vi "Current Waveform Editor.vi"() -> ()   [LabVIEW 2017]
uses:
  <vilib>/Waveform/WDTOps.llb/WDT Append Waveforms DBL.vi
  <vilib>/Waveform/WDTFileIO.llb/ Write Waveform to File.vi
  <vilib>/Waveform/WDTOps.llb/WDT Waveform Duration DBL.vi
panel:
  in  "Load 4":bool
  out "Estimate Time 2":dbl caption="Estimate Time" format="%#_4p (H)"
  out "Estimate Time":dbl format="%#_4p (H)"
  in  "Battery":dbl=310.0 format="%#_6p(mAh)"
  out "Max 3":dbl
  out "Record#":i32
  out "dt":dbl
  out "File_duration(s)":dbl
  in  "Load_Org":bool
  out "Min_F_File":dbl
  out "Max_F_FILE":dbl
  out "Min":dbl
  out "Max":dbl
  out "Min File":path
  out "Max_file":path
  out "Total Samples (20KS)":dbl format="%#_9g"
  out "Total_Duration":dbl
  out "X2_FILE#":dbl
  out "X1_FILE#":dbl
  out "#WF IN File":i32[](array[numeric])
  out "X2_20KS_FILE#":dbl
  out "X1_20KS_FILE#":dbl
  out "X2_20KS":dbl
  out "X1_20KS":dbl
  out "Duration":dbl
  out "File_list":path[](array[path])
  in  "Load 3":bool
  out "Loop ?":i32
  out "selected path 2":path caption="selected path"
  out "selected path":path
  out "Sample Rate 2":dbl caption="Sample Rate" format="%#.6pS/s"
  in  "Load 2":bool
  out "Waveform_main 2":waveform(dbl)(graph)
  out "Avg (mA) 2":dbl caption="Avg (mA)"
  out "Minutes 2":u32 caption="Total Time" format="%<%H:%M:%S>t"
  in  "Save 2":bool
  in  "Center 2":bool
  in  "ZOOM M1M2 2":bool
  in  "Clear Graph 2":bool
  out "Min 2":dbl
  in  "Orginal 2":bool
  out "Total Time":u32 format="%<%H:%M:%S>t"
  out "Avg (mA)":dbl
  out "Sample Rate":dbl format="%#.6pS/s"
  in  "Save":bool
  in  "Load":bool
  in  "Orginal":bool
  in  "Clear Graph":bool
  in  "ZOOM M1M2":bool
  in  "stop":bool
  in  "Center":bool
  out "Waveform_main":waveform(dbl)(graph)
  out "Boolean":bool
  in  "uA_bank0":dbl=1.5 format="%#_13g"
  # "Current Waveform Editor V1.0"
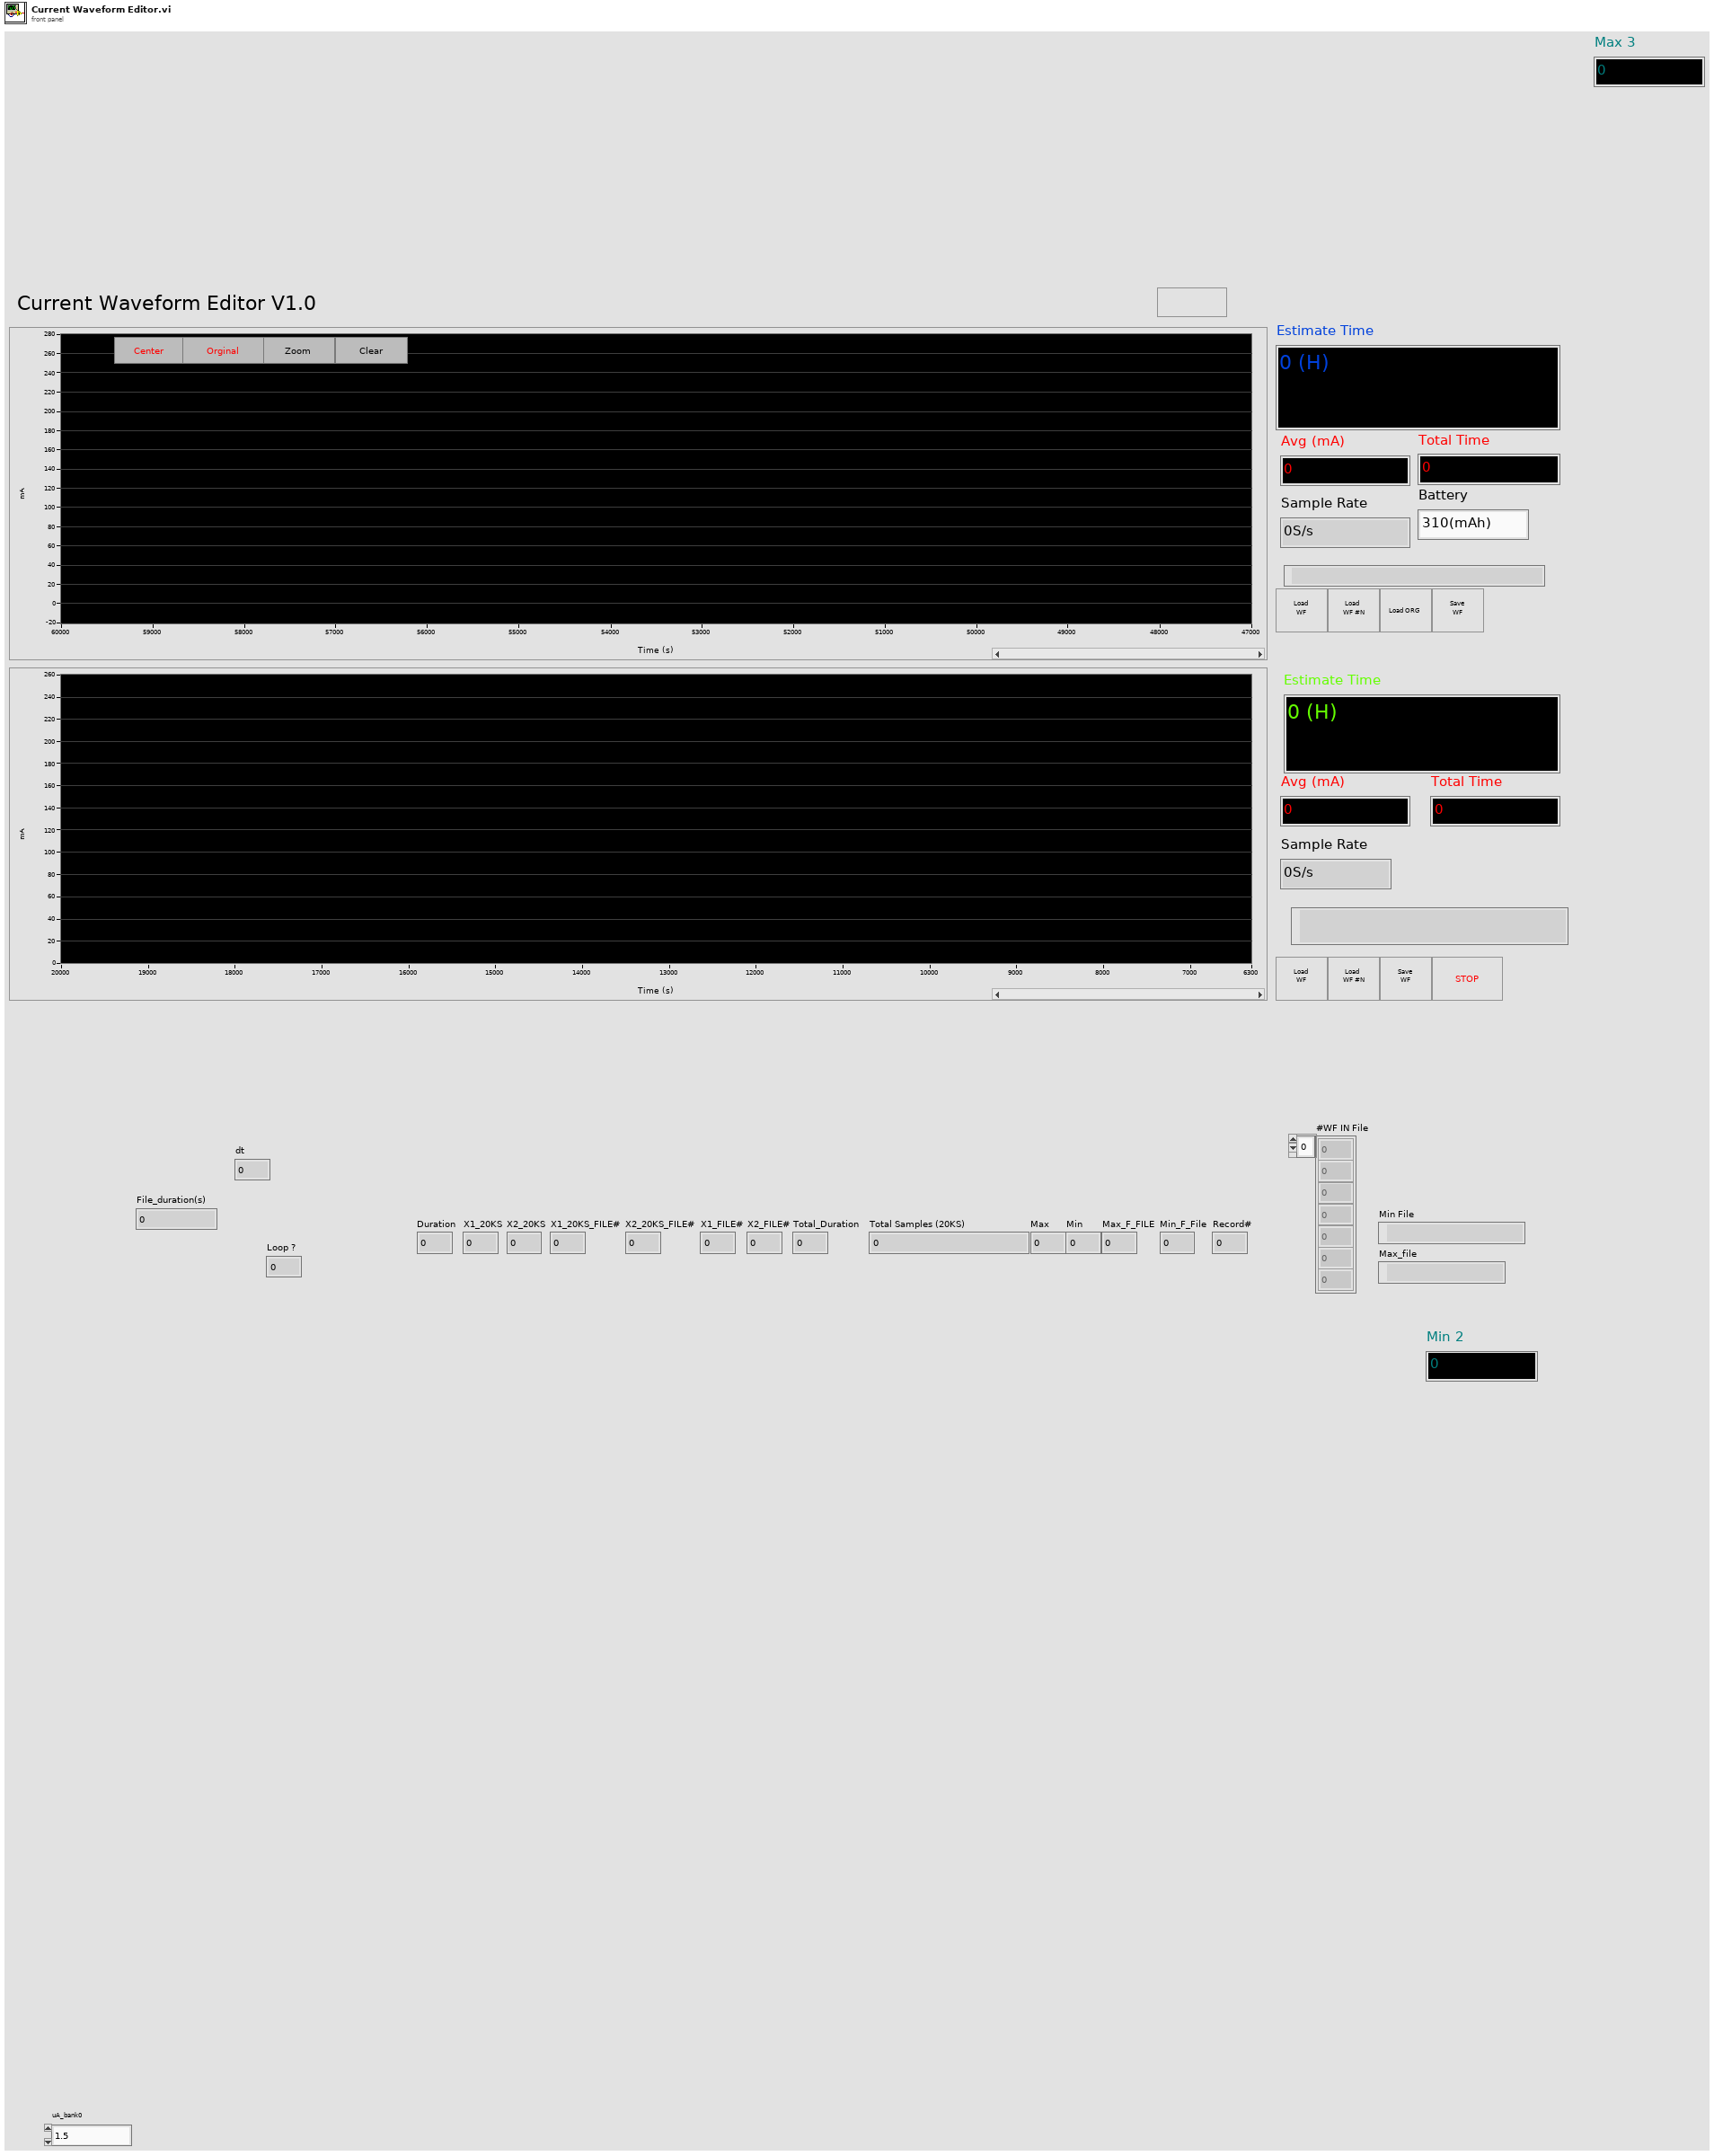
[diagram p1: front panel]
types:
  T1 = typedef "LVCursorListTypeDef.ctl" = cluster{"Name":string, "Color":u32, "Style":u8, "Point Style":u8, "Name Visible":bool, "Allow Drag":bool, "Cursor Mode":u32, "Plot":i32, "Index":i32, "Position":cluster{"X":dbl, "Y":dbl}, "X Scale":u32, "Y Scale":u32, "Watch Plots":i32[], "Watch All Plots":bool, "Plot Area":i32, "Label Offset":cluster{"X":dbl, "Y":dbl}}[]
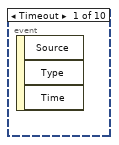
[diagram p2: hidden frame]
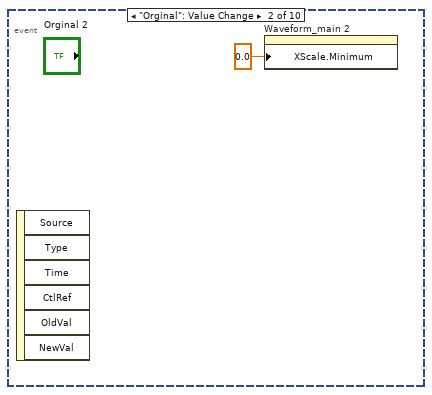
[diagram p3: hidden frame]
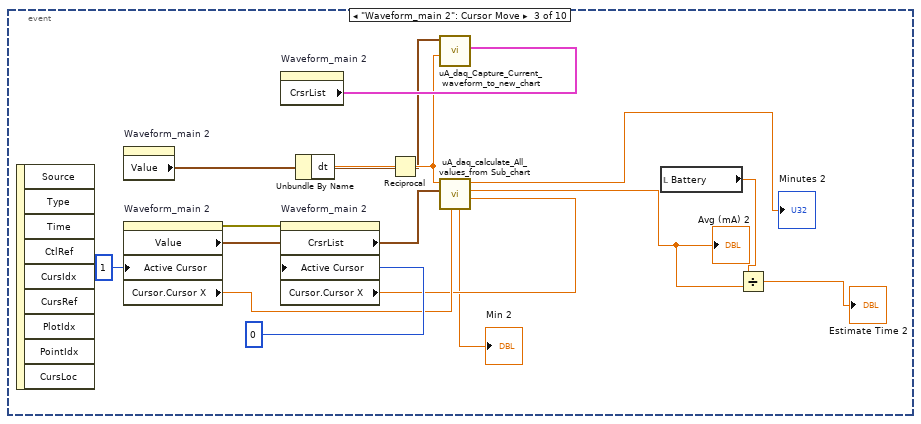
[diagram p4: hidden frame]
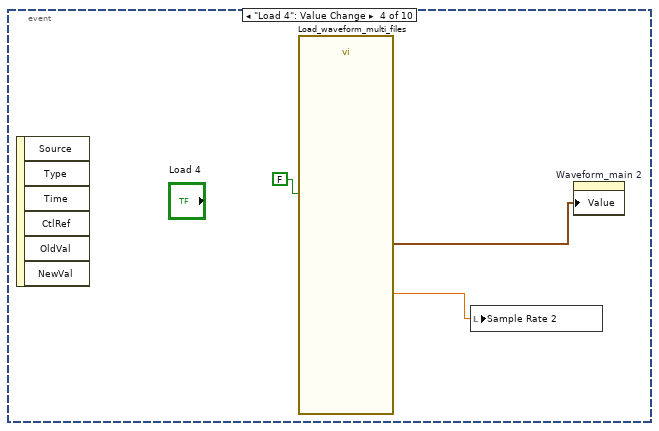
[diagram p5: hidden frame]
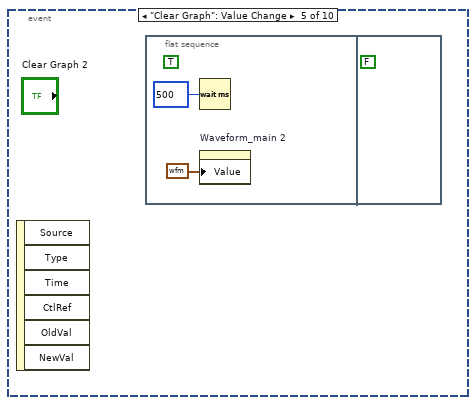
[diagram p6: hidden frame]
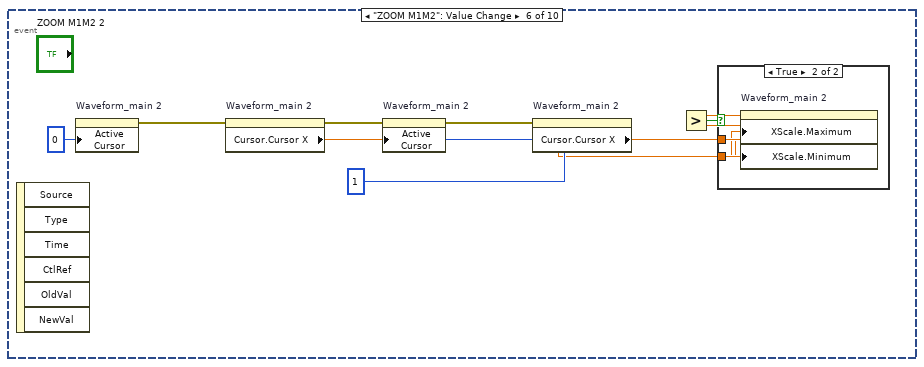
[diagram p7: hidden frame]
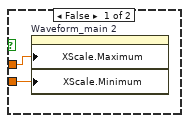
[diagram p8: hidden frame]
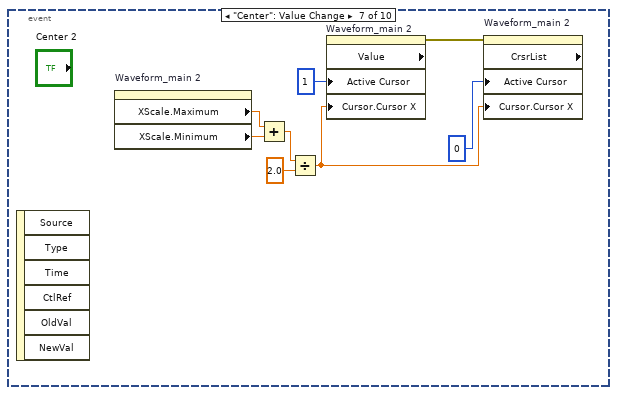
[diagram p9: hidden frame]
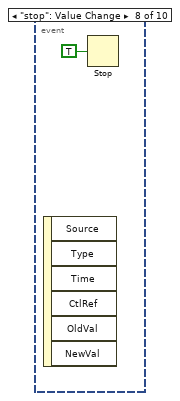
[diagram p10: hidden frame]
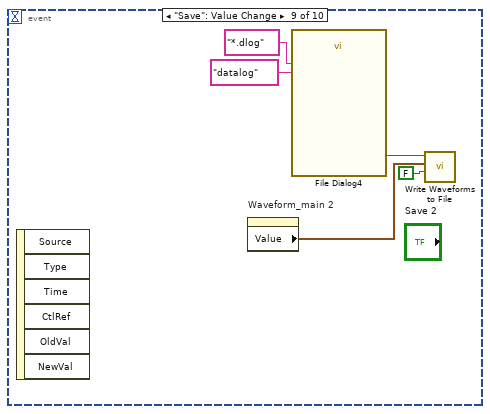
[diagram p11: hidden frame]
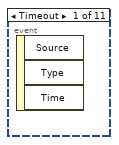
[diagram p12: hidden frame]
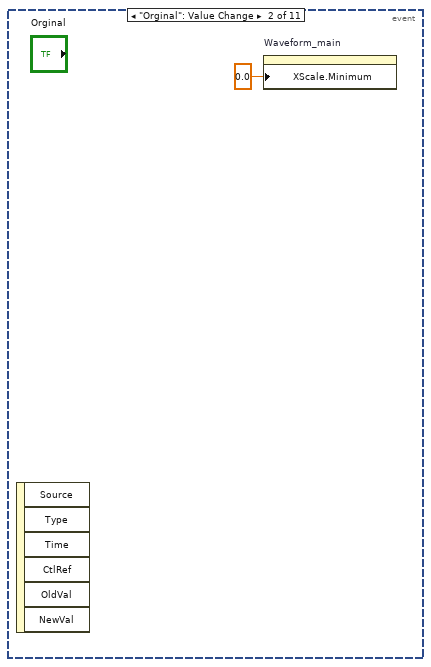
[diagram p13: hidden frame]
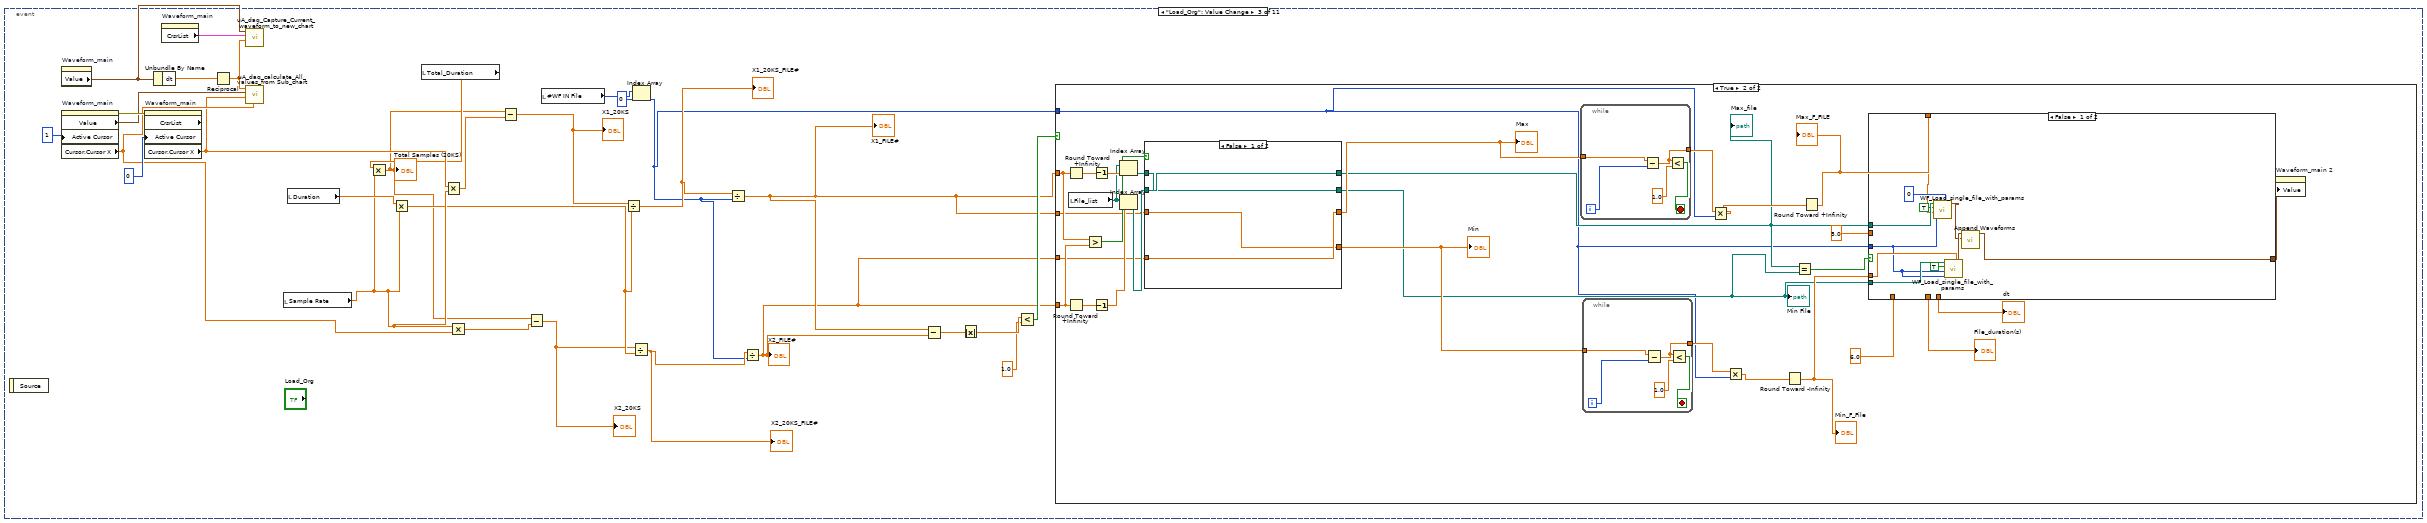
[diagram p14: hidden frame]
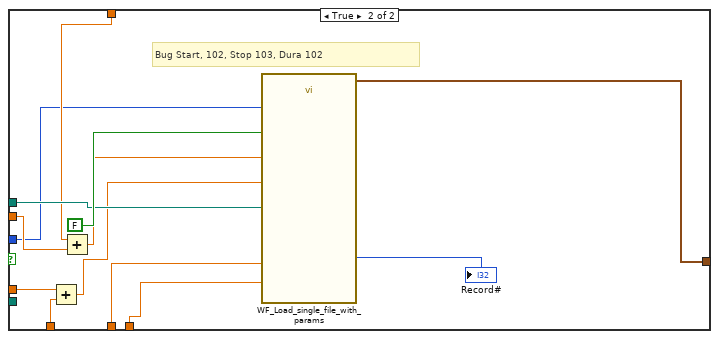
[diagram p16: hidden frame]
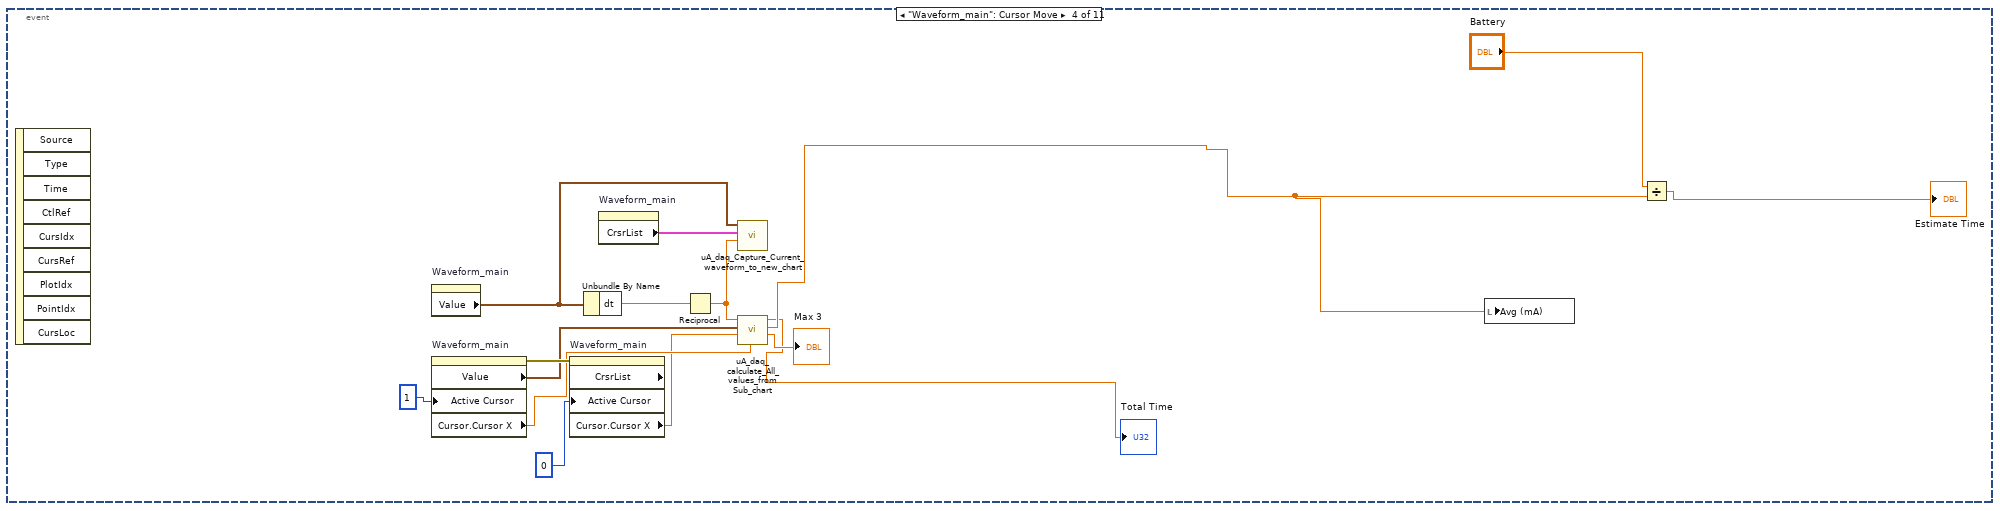
[diagram p18: hidden frame]
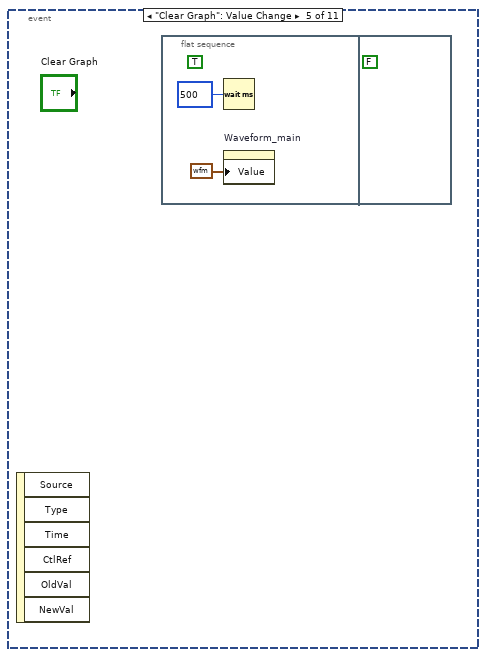
[diagram p19: hidden frame]
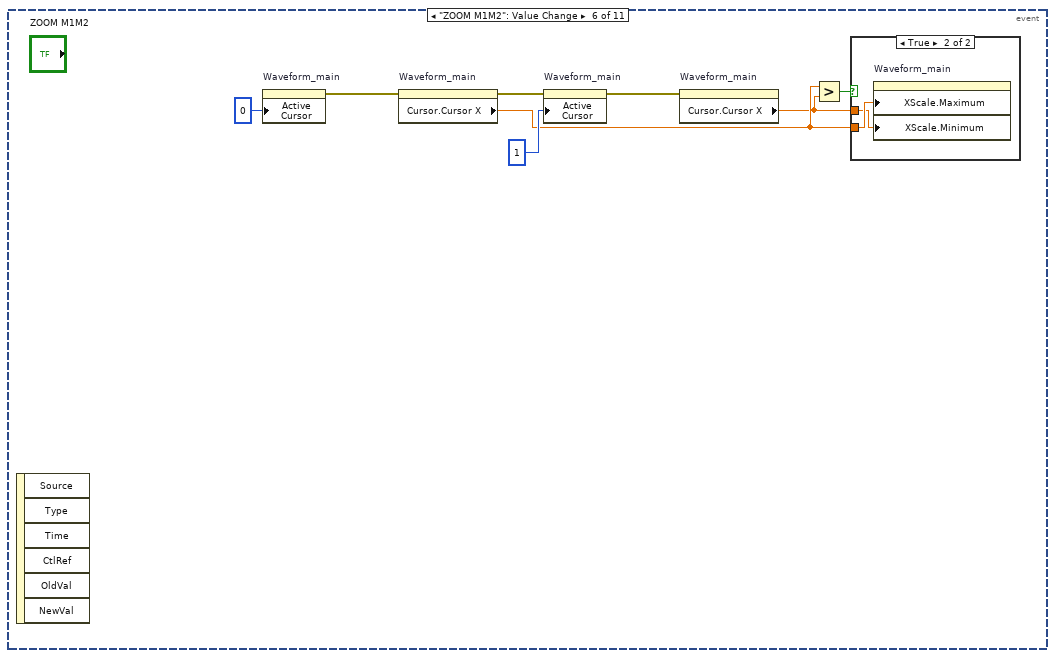
[diagram p20: hidden frame]
diagram:
  n1 = while {
    stop <- FALSE stop-if-true
    n2 = event shown="[9] \"Load\": Value Change" {
      selector: _ -> [_ _ _ _ _ _ _ _ _ _ _]
      dyn-events: _ -> [_ _ _ _ _ _ _ _ _ _ _]
      timeout: _ -> [_ _ _ _ _ _ _ _ _ _ _]
      event Timeout {
        n3 = event-data() -> ()  [unwired: 1 in, 3 out]
      }
      event "Orginal": Value Change {
        n4 = event-data() -> ()  [unwired: 1 in, 6 out]
        n5 = property on="Waveform_main" class="WFGraph (strict)"("XScale.Minimum"=0.0 ("X Scale.Range:Minimum")) -> ()  [unwired: 2 in, 2 out]
      }
      event "Load_Org": Value Change {
        n6 = event-data() -> ()  [unwired: 1 in, 1 out]
        n7 = property on="Waveform_main" class="WFGraph (strict)"() -> ("Value"=w25:waveform(dbl))  [unwired: 2 in, 2 out]
        n8 = property on="Waveform_main" class="WFGraph (strict)"("Active Cursor"=u32 1) -> (error out=w29:errorcluster, "Value"=w28:waveform(dbl), "Cursor.Cursor X"=w23:dbl)  [unwired: 2 in, 1 out]
        n9 = property on="Waveform_main" class="WFGraph (strict)" props=["CrsrList", "Active Cursor", "Cursor", "Cursor X"](error in=w29, "Active Cursor"=u32 0) -> ("Cursor.Cursor X"=w22:dbl)  [unwired: 1 in, 3 out]
        n10 = Unbundle By Name(w25) -> ("dt"=w27:dbl)
        n11 = property on="Waveform_main" class="WFGraph (strict)"() -> ("CrsrList"=w32:T1)  [unwired: 2 in, 2 out]
        n12 = Reciprocal(x=w27) -> (1/x=w26:dbl)
        n13 = call "uA_daq_Capture_Current_waveform_to_new_chart.vi"("Sample rate"=w26, "CrsrList"=w32, "Waveform_main"=w25) -> ()  [unwired: 6 in, 3 out]
        n14 = call "uA_daq_calculate_All_values_from Sub_chart.vi"("Cursor.Cursor X 2"=w23, "Cursor.Cursor X"=w22, "Value"=w28, "Sample rate"=w26) -> ()  [unwired: 3 in, 5 out]
        n15 = local read "Sample Rate"() -> (w21:dbl)
        n16 = local read "Duration"() -> (w24:dbl)
        n17 = Multiply(x=w24, y=w21) -> (x*y=w20:dbl)
        n18 = local read "Total_Duration"() -> (w14:dbl)
        n19 = Multiply(x=w14, y=w21) -> (x*y=w11:dbl)
        "Total Samples (20KS)" <- w11
        n20 = Multiply(x=w22, y=w21) -> (x*y=w16:dbl)
        n21 = Multiply(x=w21, y=w23) -> (x*y=w13:dbl)
        n22 = Subtract(x=w11, y=w16) -> (x-y=w15:dbl)
        "X1_20KS" <- w15
        n23 = Subtract(x=w11, y=w13) -> (x-y=w12:dbl)
        "X2_20KS" <- w12
        n24 = local read "#WF IN File"() -> (w18:i32[])
        n25 = Divide(x=w15, y=w20) -> (x/y=w6:dbl)
        "X1_20KS_FILE#" <- w6
        n26 = Index Array(array=w18, index=0) -> (element=w3:i32)
        n27 = Divide(x=w12, y=w20) -> (x/y=w17:dbl)
        "X2_20KS_FILE#" <- w17
        n28 = Divide(x=w6, y=w3) -> (x/y=w5:dbl)
        "X1_FILE#" <- w5
        n29 = Divide(x=w17, y=w3) -> (x/y=w4:dbl)
        "X2_FILE#" <- w4
        n30 = Subtract(x=w5, y=w4) -> (x-y=w10:dbl)
        n31 = Absolute Value(x=w10) -> (abs(x)=w9:dbl)
        n32 = Less?(x=w9, y=1.0) -> (x < y?=w7:bool)
        n33 = case shown="True" w7 {
          tunnel: w5 -> [_ w61]
          tunnel: w4 -> [_ w60]
          tunnel: w5 -> [_ w51]
          tunnel: w4 -> [_ w50]
          tunnel: w3 -> [_ w36]
          frame False {
          }
          frame True {
            n34 = Round Toward +Infinity(x=w61) -> (ceil(x): smallest int >= x=w59:dbl)
            n35 = Round Toward +Infinity(x=w60) -> (ceil(x): smallest int >= x=w58:dbl)
            n36 = local read "File_list"() -> (w55:path[])
            n37 = Greater?(x=w61, y=w60) -> (0:w54:bool)
            n38 = Decrement(x=w59) -> (x-1=w57:dbl)
            n39 = Decrement(x=w58) -> (x-1=w56:dbl)
            n40 = Index Array(array=w55, index=w57) -> (element=w53:path)
            n41 = Index Array(array=w55, index=w56) -> (element=w52:path)
            n42 = case shown="False" w54 {
              tunnel: w53 -> [w98 w103]
              tunnel: [w99 w103] -> w42
              tunnel: w52 -> [w99 w102]
              tunnel: [w98 w102] -> w37
              tunnel: w51 -> [w96 w101]
              tunnel: [w97 w101] -> w49
              tunnel: w50 -> [w97 w100]
              tunnel: [w96 w100] -> w48
              frame False {
              }
              frame True {
              }
            }
            "Max_file" <- w42
            "Min File" <- w37
            "Max" <- w49
            "Min" <- w48
            n43 = while {
              tunnel: w49 -> [w95]
              tunnel: [w91] -> w46
              i -> [w94]
              stop <- w92 stop-if-true
              n44 = Subtract(x=w95, y=w94) -> (x-y=w91:dbl)
              n45 = Less?(x=w91, y=1.0) -> (x < y?=w92:bool)
            }
            n46 = while {
              tunnel: w48 -> [w90]
              tunnel: [w86] -> w47
              i -> [w89]
              stop <- w87 stop-if-true
              n47 = Subtract(x=w90, y=w89) -> (x-y=w86:dbl)
              n48 = Less?(x=w86, y=1.0) -> (x < y?=w87:bool)
            }
            n49 = Multiply(x=w46, y=w36) -> (x*y=w45:dbl)
            n50 = Multiply(x=w47, y=w36) -> (x*y=w44:dbl)
            n51 = Round Toward -Infinity(1:w44) -> (0:w41:dbl)
            "Min_F_File" <- w41
            n52 = Equal?(x=w42, y=w37) -> (x = y?=w43:bool)
            n53 = Round Toward +Infinity(x=w45) -> (ceil(x): smallest int >= x=w40:dbl)
            "Max_F_FILE" <- w40
            n54 = case shown="False" w43 {
              tunnel: w40 -> [w67 w80]
              tunnel: w42 -> [w70 w84]
              tunnel: w41 -> [w72 w77]
              tunnel: [w69 w83] -> w33
              tunnel: [_ w82] -> w39
              tunnel: [_ w81] -> w38
              tunnel: w37 -> [w71 _]
              tunnel: w36 -> [w64 w73]
              tunnel: 5.0 ("y") -> [_ w79]
              tunnel: 6.0 ("y 2") -> [_ w76]
              frame False {
                n55 = call "WF_Load_single_file_with_params.vi"("Record#_START"=0, "N of Record"=w64, "Record# STOP"=w67, "Enable limit = True"=TRUE, "WF_FILE_IN"=w70) -> ("Waveform"=w65:waveform(dbl))  [unwired: 3 in, 3 out]
                n56 = call "WF_Load_single_file_with_params.vi"("Record#_START"=w72, "N of Record"=w64, "Record# STOP"=w64, "Enable limit = True"=TRUE, "WF_FILE_IN"=w71) -> ("Waveform"=w66:waveform(dbl))  [unwired: 3 in, 3 out]
                n57 = call-poly <vilib>:"Append Waveforms.vi"("waveform B"=w65, "waveform A"=w66) -> ("waveform out"=w69:waveform(dbl))  [unwired: 8 in, 1 out]
              }
              frame True {
                # "Bug Start, 102, Stop 103, Dura 102"
                n58 = Add(x=w77, y=w76) -> (x+y=w75:dbl)
                n59 = Add(x=w80, y=w79) -> (x+y=w78:dbl)
                n60 = call "WF_Load_single_file_with_params.vi"("Record#_START"=w75, "N of Record"=w73, "Record# STOP"=w78, "Enable limit = True"=FALSE, "WF_FILE_IN"=w84) -> ("Sampling rate"=w81:dbl, "Record#"=→"Record#":i32, "Waveform"=w83:waveform(dbl), "File_duration(s)"=w82:dbl)  [unwired: 3 in]
              }
            }
            "File_duration(s)" <- w39
            "dt" <- w38
            n61 = property on="Waveform_main 2" class="WFGraph (strict)"("Value"=w33) -> ()  [unwired: 2 in, 2 out]
          }
        }
      }
      event "Waveform_main": Cursor Move {
        n62 = event-data() -> ()  [unwired: 1 in, 9 out]
        n63 = property on="Waveform_main" class="WFGraph (strict)"() -> ("Value"=w112:waveform(dbl))  [unwired: 2 in, 2 out]
        n64 = property on="Waveform_main" class="WFGraph (strict)"("Active Cursor"=u32 1) -> (error out=w116:errorcluster, "Value"=w115:waveform(dbl), "Cursor.Cursor X"=w111:dbl)  [unwired: 2 in, 1 out]
        n65 = property on="Waveform_main" class="WFGraph (strict)" props=["CrsrList", "Active Cursor", "Cursor", "Cursor X"](error in=w116, "Active Cursor"=u32 0) -> ("Cursor.Cursor X"=w110:dbl)  [unwired: 1 in, 3 out]
        n66 = Unbundle By Name(w112) -> ("dt"=w114:dbl)
        n67 = property on="Waveform_main" class="WFGraph (strict)"() -> ("CrsrList"=w117:T1)  [unwired: 2 in, 2 out]
        n68 = Reciprocal(x=w114) -> (1/x=w113:dbl)
        n69 = call "uA_daq_Capture_Current_waveform_to_new_chart.vi"("Sample rate"=w113, "CrsrList"=w117, "Waveform_main"=w112) -> ()  [unwired: 6 in, 3 out]
        n70 = call "uA_daq_calculate_All_values_from Sub_chart.vi"("Cursor.Cursor X 2"=w111, "Cursor.Cursor X"=w110, "Value"=w115, "Sample rate"=w113) -> ("Max value"=→"Max 3":dbl, "Average"=w105:dbl, "Delta(s)"=→"Total Time":sgl)  [unwired: 3 in, 2 out]
        n71 = local write "Avg (mA)"(w105) -> ()
        n72 = Divide(x="Battery", y=w105) -> (x/y=→"Estimate Time":dbl)
      }
      event "Clear Graph": Value Change {
        n73 = event-data() -> ()  [unwired: 1 in, 6 out]
        n74 = flat-sequence {
          frame #0 {
            (unwired) TRUE ("Clear")
            n75 = Wait (ms)(milliseconds to wait=u32 500) -> ()  [unwired: 1 out]
            n76 = property on="Waveform_main" class="WFGraph (strict)"("Value"=waveform(sgl) {"t0"=timestamp(0 s since 1904-01-01), "dt"=1.0, "Y"=[]} ("Waveform_main")) -> ()  [unwired: 2 in, 2 out]
          }
          frame #1 {
            (unwired) FALSE ("Clear")
          }
        }
      }
      event "ZOOM M1M2": Value Change {
        n77 = event-data() -> ()  [unwired: 1 in, 6 out]
        n78 = property on="Waveform_main" class="WFGraph (strict)"("Active Cursor"=u32 0) -> (error out=w127:errorcluster)  [unwired: 2 in, 1 out]
        n79 = property on="Waveform_main" class="WFGraph (strict)"(error in=w127) -> (error out=w124:errorcluster, "Cursor.Cursor X"=w122:dbl)  [unwired: 1 in, 1 out]
        n80 = property on="Waveform_main" class="WFGraph (strict)"(error in=w124, "Active Cursor"=u32 1) -> (error out=w126:errorcluster)  [unwired: 1 in, 1 out]
        n81 = property on="Waveform_main" class="WFGraph (strict)"(error in=w126) -> ("Cursor.Cursor X"=w121:dbl)  [unwired: 1 in, 2 out]
        n82 = Greater?(x=w122, y=w121) -> (0:w123:bool)
        n83 = case shown="True" w123 {
          tunnel: w122 -> [w130 w132]
          tunnel: w121 -> [w129 w131]
          frame False {
            n84 = property on="Waveform_main" class="WFGraph (strict)"("XScale.Maximum"=w129, "XScale.Minimum"=w130) -> ()  [unwired: 2 in, 2 out]
          }
          frame True {
            n85 = property on="Waveform_main" class="WFGraph (strict)"("XScale.Maximum"=w132, "XScale.Minimum"=w131) -> ()  [unwired: 2 in, 2 out]
          }
        }
      }
      event "Center": Value Change {
        n86 = event-data() -> ()  [unwired: 1 in, 6 out]
        n87 = property on="Waveform_main" class="WFGraph (strict)"() -> ("XScale.Maximum"=w137:dbl, "XScale.Minimum"=w136:dbl)  [unwired: 2 in, 2 out]
        n88 = Add(x=w137, y=w136) -> (x+y=w135:dbl)
        n89 = Divide(x=w135, y=2.0) -> (x/y=w133:dbl)
        n90 = property on="Waveform_main" class="WFGraph (strict)" props=["Value", "Active Cursor", "Cursor", "Cursor X"]("Active Cursor"=u32 1, "Cursor.Cursor X"=w133) -> (error out=w138:errorcluster)  [unwired: 2 in, 2 out]
        n91 = property on="Waveform_main" class="WFGraph (strict)" props=["CrsrList", "Active Cursor", "Cursor", "Cursor X"](error in=w138, "Active Cursor"=u32 0, "Cursor.Cursor X"=w133) -> ()  [unwired: 1 in, 3 out]
      }
      event "stop": Value Change {
        n92 = event-data() -> ()  [unwired: 1 in, 6 out]
        n93 = Stop(stop? (T)=TRUE) -> ()
      }
      event "Save": Value Change {
        n94 = event-data() -> ()  [unwired: 1 in, 6 out]
        n95 = call "File Dialog"("pattern (all files)"="*.dlog", "pattern label"="datalog") -> ("selected path"=w146:path)  [unwired: 10 in, 3 out]
        n96 = property on="Waveform_main" class="WFGraph (strict)"() -> ("Value"=w142:waveform(dbl))  [unwired: 2 in, 2 out]
        n97 = call-poly <vilib>:"Write Waveforms to File.vi"("append to file? (new file:F)"=FALSE, "waveform"=w142, "file path (dialog if empty)"=w146) -> ()  [unwired: 7 in, 2 out]
      }
      event "Load": Value Change {
        (unwired) 1000 ("N 2")
        w154 = 60.0 ("y")
        n98 = event-data() -> ()  [unwired: 1 in, 6 out]
        n99 = call "Load_waveform_file.vi"("N"=1000 ("N 2"), "Enable limit = True"=FALSE) -> ("Loop ?"=→"Loop ?":i32, "selected path"=→"selected path":path, "first waveform in record"=w148:waveform(dbl), "Sample_Rate"=w147:dbl)  [unwired: 6 in]
        n100 = Unbundle By Name(w148) -> ("Y"=w159:dbl[])  [unwired: 1 out]
        n101 = call-poly <vilib>:"Waveform Duration.vi"("waveform in"=w148) -> ("duration"=w155:dbl)  [unwired: 8 in, 2 out]
        n102 = Add Array Elements(numeric array=w159) -> (sum=w158:dbl)
        n103 = Divide(x=w155, y=w154) -> (x/y=w153:dbl)
        n104 = Array Size(array=w159) -> (size(s)=w157:i32)
        n105 = Divide(x=w158, y=w157) -> (x/y=→"Avg (mA)":dbl)
        n106 = Divide(x=w153, y=w154) -> ()  [unwired: 1 out]
        n107 = property on="Waveform_main" class="WFGraph (strict)"("Value"=w148) -> ()  [unwired: 2 in, 2 out]
        n108 = local write "Sample Rate"(w147) -> ()
      }
      event "Load 3": Value Change {
        n109 = event-data() -> ()  [unwired: 1 in, 6 out]
        n110 = call "Load_waveform_multi_files.vi"("Enable limit = True"=FALSE) -> ("File_list"=→"File_list":path[], "Total_Duration"=→"Total_Duration":dbl, "first waveform in record"=→"Waveform_main":waveform(dbl), "#WF IN File"=→"#WF IN File":i32[], "Duration"=→"Duration":dbl, "Sample rate"=→"Sample Rate":dbl)  [unwired: 11 in, 2 out]
      }
    }
  }
  n111 = while {
    stop <- FALSE stop-if-true
    n112 = event shown="[9] \"Load 2\": Value Change" {
      selector: _ -> [_ _ _ _ _ _ _ _ _ _]
      dyn-events: _ -> [_ _ _ _ _ _ _ _ _ _]
      timeout: _ -> [_ _ _ _ _ _ _ _ _ _]
      event Timeout {
        n113 = event-data() -> ()  [unwired: 1 in, 3 out]
      }
      event "Orginal": Value Change {
        n114 = event-data() -> ()  [unwired: 1 in, 6 out]
        n115 = property on="Waveform_main 2" class="WFGraph (strict)"("XScale.Minimum"=0.0 ("X Scale.Range:Minimum")) -> ()  [unwired: 2 in, 2 out]
      }
      event "Waveform_main 2": Cursor Move {
        n116 = event-data() -> ()  [unwired: 1 in, 9 out]
        n117 = property on="Waveform_main 2" class="WFGraph (strict)"() -> ("Value"=w173:waveform(dbl))  [unwired: 2 in, 2 out]
        n118 = property on="Waveform_main 2" class="WFGraph (strict)"("Active Cursor"=u32 1) -> (error out=w178:errorcluster, "Value"=w177:waveform(dbl), "Cursor.Cursor X"=w180:dbl)  [unwired: 2 in, 1 out]
        n119 = property on="Waveform_main 2" class="WFGraph (strict)"() -> ("CrsrList"=w183:T1)  [unwired: 2 in, 2 out]
        n120 = property on="Waveform_main 2" class="WFGraph (strict)" props=["CrsrList", "Active Cursor", "Cursor", "Cursor X"](error in=w178, "Active Cursor"=u32 0) -> ("Cursor.Cursor X"=w179:dbl)  [unwired: 1 in, 3 out]
        n121 = Unbundle By Name(w173) -> ("dt"=w175:dbl)
        n122 = Reciprocal(x=w175) -> (1/x=w174:dbl)
        n123 = call "uA_daq_Capture_Current_waveform_to_new_chart.vi"("Sample rate"=w174, "CrsrList"=w183, "Waveform_main"=w173) -> ()  [unwired: 6 in, 3 out]
        n124 = call "uA_daq_calculate_All_values_from Sub_chart.vi"("Cursor.Cursor X 2"=w180, "Cursor.Cursor X"=w179, "Value"=w177, "Sample rate"=w174) -> ("Average"=w170:dbl, "Delta(s)"=→"Minutes 2":sgl, "Min value"=→"Min 2":dbl)  [unwired: 3 in, 2 out]
        "Avg (mA) 2" <- w170
        n125 = local read "Battery"() -> (w171:dbl)
        n126 = Divide(x=w171, y=w170) -> (x/y=→"Estimate Time 2":dbl)
      }
      event "Load 4": Value Change {
        n127 = event-data() -> ()  [unwired: 1 in, 6 out]
        n128 = call "Load_waveform_multi_files.vi"("Enable limit = True"=FALSE) -> ("first waveform in record"=w185:waveform(dbl), "Sample rate"=w184:dbl)  [unwired: 11 in, 6 out]
        n129 = local write "Sample Rate 2"(w184) -> ()
        n130 = property on="Waveform_main 2" class="WFGraph (strict)"("Value"=w185) -> ()  [unwired: 2 in, 2 out]
      }
      event "Clear Graph": Value Change {
        n131 = event-data() -> ()  [unwired: 1 in, 6 out]
        n132 = flat-sequence {
          frame #0 {
            (unwired) TRUE ("Clear")
            n133 = Wait (ms)(milliseconds to wait=u32 500) -> ()  [unwired: 1 out]
            n134 = property on="Waveform_main 2" class="WFGraph (strict)"("Value"=waveform(sgl) {"t0"=timestamp(0 s since 1904-01-01), "dt"=1.0, "Y"=[]} ("Waveform_main")) -> ()  [unwired: 2 in, 2 out]
          }
          frame #1 {
            (unwired) FALSE ("Clear")
          }
        }
      }
      event "ZOOM M1M2": Value Change {
        n135 = event-data() -> ()  [unwired: 1 in, 6 out]
        n136 = property on="Waveform_main 2" class="WFGraph (strict)"("Active Cursor"=u32 0) -> (error out=w195:errorcluster)  [unwired: 2 in, 1 out]
        n137 = property on="Waveform_main 2" class="WFGraph (strict)"(error in=w195) -> (error out=w192:errorcluster, "Cursor.Cursor X"=w190:dbl)  [unwired: 1 in, 1 out]
        n138 = property on="Waveform_main 2" class="WFGraph (strict)"(error in=w192, "Active Cursor"=u32 1) -> (error out=w194:errorcluster)  [unwired: 1 in, 1 out]
        n139 = property on="Waveform_main 2" class="WFGraph (strict)"(error in=w194) -> ("Cursor.Cursor X"=w189:dbl)  [unwired: 1 in, 2 out]
        n140 = Greater?(x=w190, y=w189) -> (0:w191:bool)
        n141 = case shown="True" w191 {
          tunnel: w190 -> [w198 w200]
          tunnel: w189 -> [w197 w199]
          frame False {
            n142 = property on="Waveform_main 2" class="WFGraph (strict)"("XScale.Maximum"=w197, "XScale.Minimum"=w198) -> ()  [unwired: 2 in, 2 out]
          }
          frame True {
            n143 = property on="Waveform_main 2" class="WFGraph (strict)"("XScale.Maximum"=w200, "XScale.Minimum"=w199) -> ()  [unwired: 2 in, 2 out]
          }
        }
      }
      event "Center": Value Change {
        n144 = event-data() -> ()  [unwired: 1 in, 6 out]
        n145 = property on="Waveform_main 2" class="WFGraph (strict)"() -> ("XScale.Maximum"=w205:dbl, "XScale.Minimum"=w204:dbl)  [unwired: 2 in, 2 out]
        n146 = Add(x=w205, y=w204) -> (x+y=w203:dbl)
        n147 = Divide(x=w203, y=2.0) -> (x/y=w201:dbl)
        n148 = property on="Waveform_main 2" class="WFGraph (strict)" props=["Value", "Active Cursor", "Cursor", "Cursor X"]("Active Cursor"=u32 1, "Cursor.Cursor X"=w201) -> (error out=w206:errorcluster)  [unwired: 2 in, 2 out]
        n149 = property on="Waveform_main 2" class="WFGraph (strict)" props=["CrsrList", "Active Cursor", "Cursor", "Cursor X"](error in=w206, "Active Cursor"=u32 0, "Cursor.Cursor X"=w201) -> ()  [unwired: 1 in, 3 out]
      }
      event "stop": Value Change {
        n150 = event-data() -> ()  [unwired: 1 in, 6 out]
        n151 = Stop(stop? (T)=TRUE) -> ()
      }
      event "Save": Value Change {
        n152 = event-data() -> ()  [unwired: 1 in, 6 out]
        n153 = property on="Waveform_main 2" class="WFGraph (strict)"() -> ("Value"=w210:waveform(dbl))  [unwired: 2 in, 2 out]
        n154 = call "File Dialog4"("pattern (all files)"="*.dlog", "pattern label"="datalog") -> ("selected path"=w214:path)  [unwired: 10 in, 3 out]
        n155 = call-poly <vilib>:"Write Waveforms to File.vi"("append to file? (new file:F)"=FALSE, "waveform"=w210, "file path (dialog if empty)"=w214) -> ()  [unwired: 7 in, 2 out]
      }
      event "Load 2": Value Change {
        w222 = 60.0 ("y")
        (unwired) FALSE ("append to file? (new file:F)")
        n156 = event-data() -> ()  [unwired: 1 in, 6 out]
        n157 = call "Load_waveform_file.vi"("N"=1000, "Enable limit = True"=FALSE) -> ("selected path"=→"selected path 2":path, "first waveform in record"=w219:waveform(dbl), "Sample_Rate"=→"Sample Rate 2":dbl)  [unwired: 6 in, 1 out]
        n158 = call "Re_sampling_1SS.vi"("Waveform_main"=w219) -> ("Waveform"=w220:waveform(dbl))  [unwired: 10 in]
        "Waveform_main 2" <- w220
        n159 = Unbundle By Name(w220) -> ("Y"=w226:dbl[])  [unwired: 1 out]
        n160 = call-poly <vilib>:"Waveform Duration.vi"("waveform in"=w220) -> ("duration"=w223:dbl)  [unwired: 8 in, 2 out]
        n161 = Add Array Elements(numeric array=w226) -> (sum=w225:dbl)
        n162 = Array Size(array=w226) -> (size(s)=w224:i32)
        n163 = Divide(x=w223, y=w222) -> (x/y=w221:dbl)
        n164 = Divide(x=w225, y=w224) -> ()  [unwired: 1 out]
        n165 = Divide(x=w221, y=w222) -> ()  [unwired: 1 out]
      }
    }
  }
